vi "U3 Read Serial Number.vi"() -> (0 "error out":errorcluster)   [LabVIEW 2021]
panel:
  in  "FirstFound":bool=TRUE
  in  "Address":string="1"
  out "Error Message":string
  out "Value Read":i32
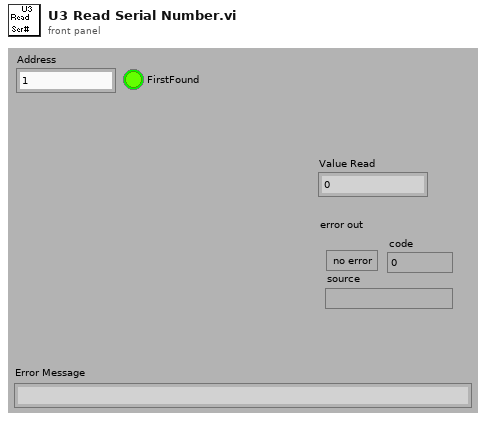
[diagram p1: front panel]
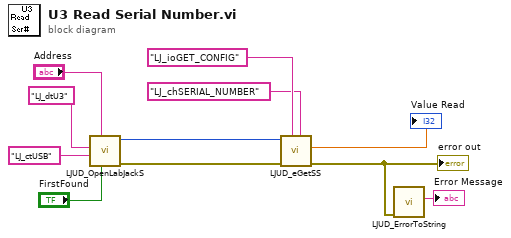
[diagram p0: block diagram]
diagram:
  n1 = call "LJUD_OpenLabJackS.vi"("FirstFound"="FirstFound", "Address"="Address", "ConnectionType"="LJ_ctUSB", "DeviceType"="LJ_dtU3") -> ("error out"=w3:errorcluster, "Handle"=w4:i32)  [unwired: 5 in, 1 out]
  n2 = call "LJUD_eGetSS.vi"("Channel"="LJ_chSERIAL_NUMBER", "IOType"="LJ_ioGET_CONFIG", "error in"=w3, "Handle In"=w4) -> ("error out"=w8:errorcluster, "Value Read"=→"Value Read":dbl)  [unwired: 5 in, 1 out]
  "error out" <- w8
  n3 = call "LJUD_ErrorToString.vi"("error in"=w8) -> ("String"=→"Error Message":string)  [unwired: 10 in]
